vi "Launch.vi"(8 "error in (no error)":errorcluster, 11 "Response Channel":refnum<class "Messenger.lvclass">) -> (0 "error out":errorcluster, 3 "Actor API out":refnum<class "Actor API.lvclass">)   [LabVIEW 2015, in "Status Window.lvclass"]
doc: "<b>Response</b> channel is used by this actor to return infomation back to the parent. Typically this input is the Request channel of the parent actor."
uses:
  Status Window.lvclass
  Re-use Libraries/Minimal Actor Framework/Actors/Base Actor/API/Actor API.lvclass
  Re-use Libraries/Minimal Actor Framework/Messaging/Messenger/Messenger.lvclass
  Re-use Libraries/Minimal Actor Framework/Actors/Base Actor/Actor/Front Panel State.ctl
  Re-use Libraries/Minimal Actor Framework/Actors/Base Actor/Actor/Actor.lvclass/Actor.ctl
  Re-use Libraries/Minimal Actor Framework/Actors/Base Actor/Actor/Actor.lvclass
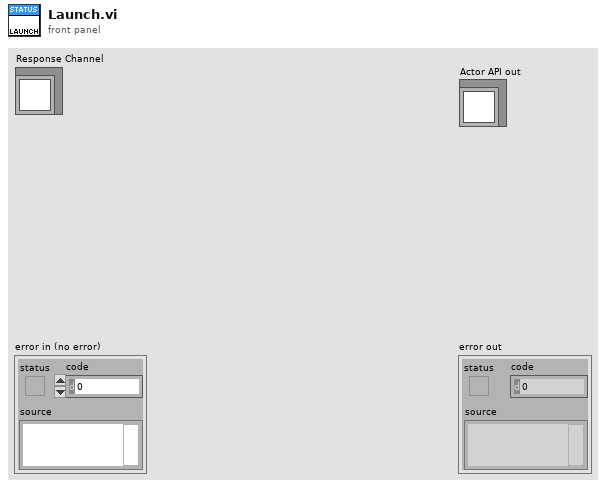
[diagram p1: front panel]
types:
  T1 = typedef "Actor.lvclass/Front Panel State.ctl" = enum32{"Invalid", "Standard", "Closed", "Hidden", "Minimized", "Maximized"}
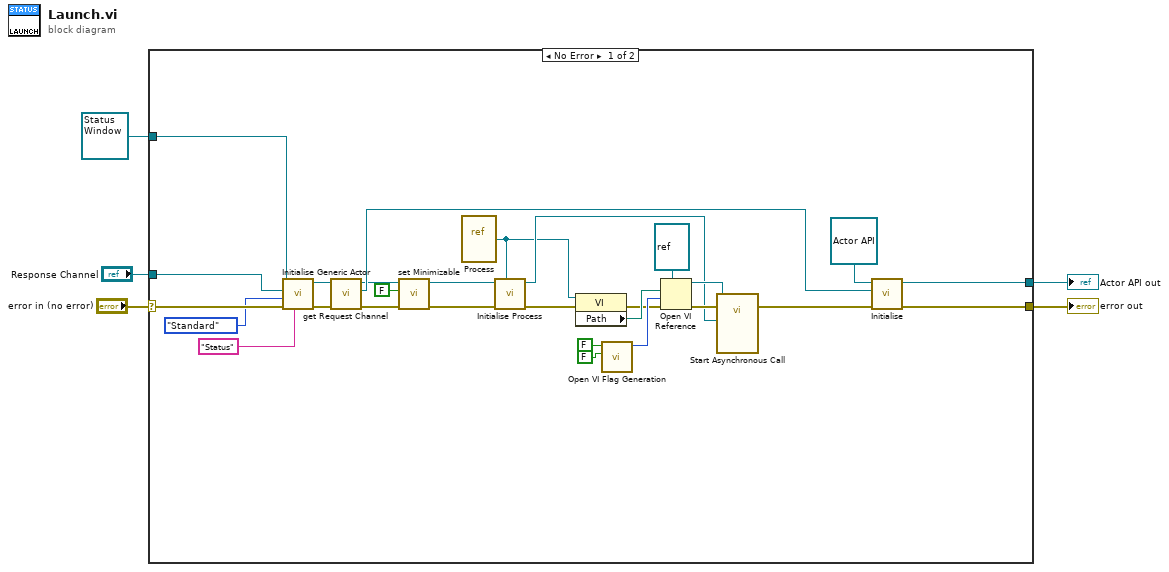
[diagram p0: block diagram]
diagram:
  n1 = case shown="No Error" "error in (no error)" {
    selector: "error in (no error)" -> [w24 w33]
    tunnel: [w21 w33] -> w5
    tunnel: [w14 _] -> w2
    tunnel: refnum<class "Status Window.lvclass"> refnum ("Worker Test 1.lvclass") -> [w23 _]
    tunnel: "Response Channel" -> [w6 _]
    frame No Error {
      n2 = call-dynamic "Initialise Generic Actor.vi"("Name"="Status", "Front Panel State"=Front_Panel_State."Standard", "Response Channel"=w6, "Actor in"=w23) -> ("Actor out"=w25:refnum<class "Status Window.lvclass">)  [unwired: 6 in, 1 out]
      n3 = call "get Request Channel.vi"("error in (no error)"=w24, "Actor in"=w25) -> ("error out"=w10:errorcluster, "Request Channel"=w26:refnum<class "Messenger.lvclass">, "Actor out"=w11:refnum<class "Status Window.lvclass">)  [unwired: 7 in]
      n4 = call "set Minimizable.vi"("error in (no error)"=w10, "Minimizable"=FALSE, "Actor in"=w11) -> ("error out"=w8:errorcluster, "Actor out"=w9:refnum<class "Status Window.lvclass">)  [unwired: 7 in]
      n5 = vi-ref "Process.vi"() -> (w15:refnum<vi>)
      n6 = call-dynamic "Initialise Process.vi"("Process"=w15, "error in (no error)"=w8, "Actor in"=w9) -> ("error out"=w16:errorcluster, "Actor out"=w17:refnum<class "Status Window.lvclass">)  [unwired: 7 in]
      n7 = property class="VI"(reference=w15, error in=w16) -> (error out=w19:errorcluster, "Path"=w20:path)  [unwired: 1 out]
      n8 = call "Open VI Flag Generation.vi"("Call And Collect (F)"=FALSE, "Re-entrant (F)"=FALSE) -> ("Flags"=w32:i32)  [unwired: 9 in]
      n9 = Open VI Reference(type specifier VI Refnum (for type only)=refnum<vi> refnum, vi path=w20, options=w32, error in (no error)=w19) -> (vi reference=w28:refnum<vi>, error out=w27:errorcluster)  [unwired: 2 in]
      n10 = call-by-ref "Start Asynchronous Call"(reference=w28, error in=w27, "Worker Test 1.lvclass"=w17) -> (error out=w12:errorcluster)  [unwired: 11 in, 1 out]
      n11 = call "Initialise.vi"("error in (no error)"=w12, "Request Channel"=w26, "Actor API in"=refnum<class "Actor API.lvclass"> refnum ("Actor API.lvclass")) -> ("error out"=w21:errorcluster, "Actor API out"=w14:refnum<class "Actor API.lvclass">)  [unwired: 7 in]
    }
    frame Error {
    }
  }
  "error out" <- w5
  "Actor API out" <- w2
